vi "create.vi"(5 "rate":dbl, 7 "name":string, 8 "error in":errorcluster, 10 "test-channel in":refnum<class "test-channel.lvclass">[](array[class]), 11 "test-group in":refnum<class "test-group.lvclass">) -> (0 "error out":errorcluster, 3 "test-group out":refnum<class "test-group.lvclass">)   [LabVIEW 2020, in "test-group.lvclass"]
uses:
  test-group.lvclass
  test-channel/test-channel.lvclass
  test-group.lvclass/test-group.ctl
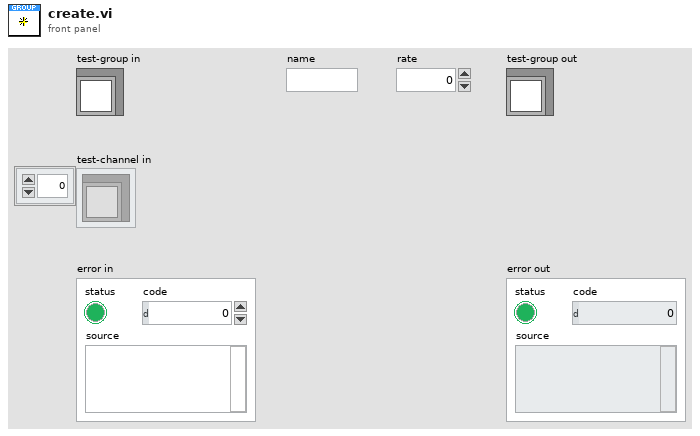
[diagram p1: front panel]
types:
  T1 = map{string, refnum<class "test-channel.lvclass">}
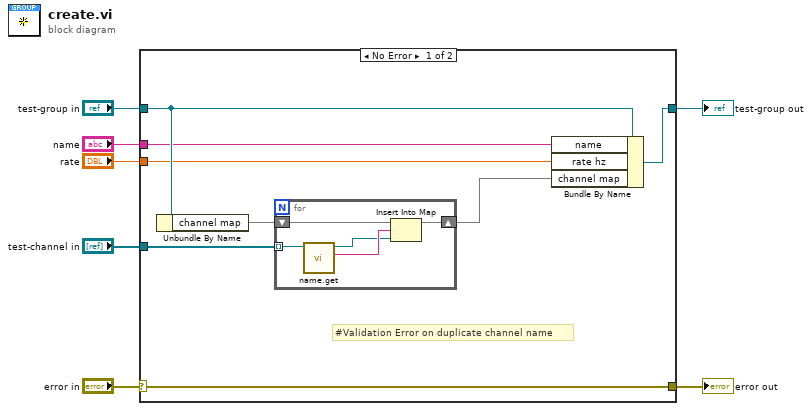
[diagram p0: block diagram]
diagram:
  n1 = case shown="No Error" "error in" {
    selector: "error in" -> [w15 w22]
    tunnel: [w15 w22] -> w6
    tunnel: [w14 w21] -> w4
    tunnel: "test-group in" -> [w11 w21]
    tunnel: "test-channel in" -> [w13 _]
    tunnel: "name" -> [w9 _]
    tunnel: "rate" -> [w8 _]
    frame No Error {
      # "#Validation Error on duplicate channel name"
      n2 = Unbundle By Name(w11) -> ("channel map"=w10:T1)
      n3 = for {
        tunnel: w13 -> [w20] mode=indexing
        shift-right: [w17] -> w12
        shift-left: w10 -> [w16]
        n4 = call "name.get.vi"("test-channel in"=w20) -> ("name"=w19:string, "test-channel out"=w18:refnum<class "test-channel.lvclass">)  [unwired: 9 in]
        n5 = Insert Into Map(map in=w16, key=w19, value=w18) -> (map out=w17:T1)  [unwired: 2 out]
      }
      n6 = Bundle By Name(cluster=w11, "name"=w9, "rate hz"=w8, "channel map"=w12) -> (w14:refnum<class "test-group.lvclass">)
    }
    frame Error {
    }
  }
  "error out" <- w6
  "test-group out" <- w4
